vi "Scoring.vi"(4 "Target Up?":bool, 7 "Cluster In":T1, 8 "Hit?":bool, 9 "Falling Edge":bool, 10 "FallingEdge":u32, 11 "RisingEdge":u32) -> (1 "Combo":u32, 2 "Live Score":u32, 3 "Cluster Out":T1)   [LabVIEW 2022 SP3]
uses:
  ShargTypeDef.ctl
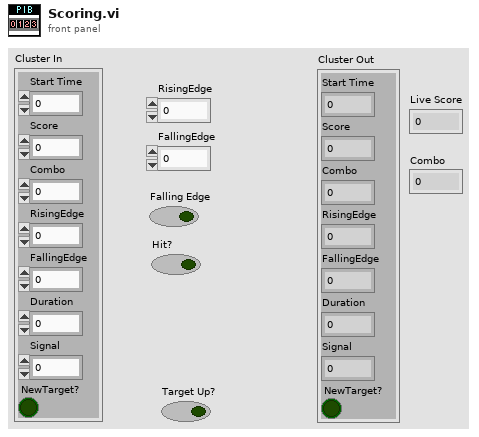
[diagram p1: front panel]
types:
  T1 = typedef "ShargTypeDef.ctl" = cluster{"Start Time":u32, "Score":u32, "Combo":u32, "RisingEdge":u32, "FallingEdge":u32, "Duration":u32, "Signal":i16, "NewTarget?":bool}
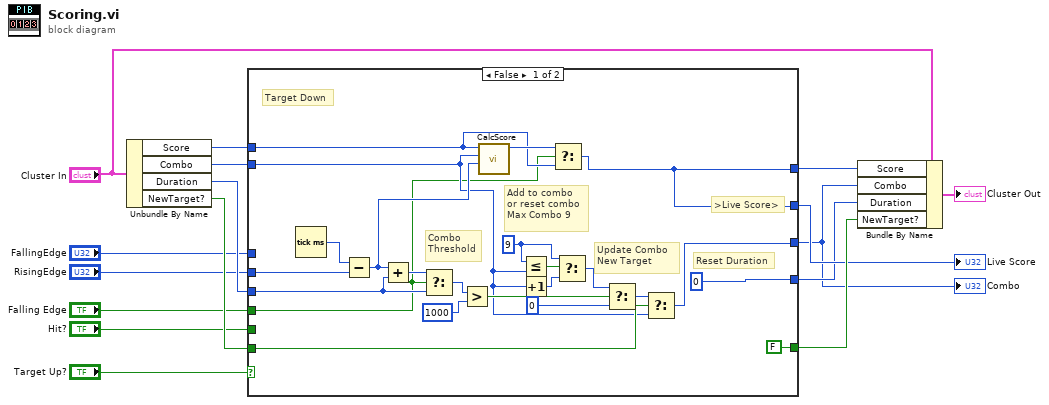
[diagram p0: block diagram]
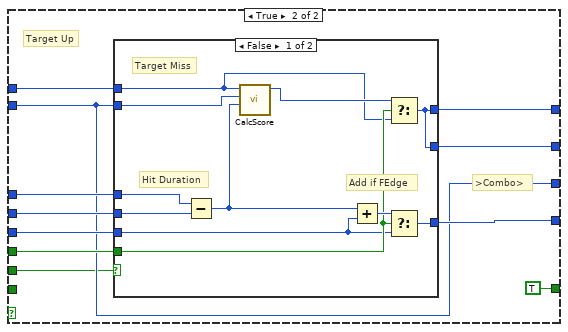
[diagram p2: hidden frame]
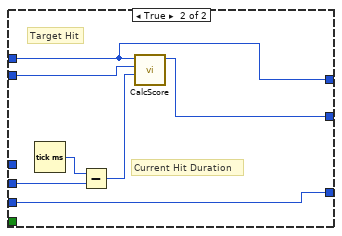
[diagram p3: hidden frame]
diagram:
  n1 = Unbundle By Name("Cluster In") -> ("Score"=w8:u32, "Combo"=w9:u32, "Duration"=w10:u32, "NewTarget?"=w11:bool)
  n2 = case shown="False" "Target Up?" {
    tunnel: "Hit?" -> [_ w40]
    tunnel: "RisingEdge" -> [w31 w45]
    tunnel: "FallingEdge" -> [_ w44]
    tunnel: w10 -> [w18 w43]
    tunnel: [u32 0 ("Duration") w50] -> w14
    tunnel: "Falling Edge" -> [w17 w49]
    tunnel: w9 -> [w25 w42]
    tunnel: [w35 w42] -> w13
    tunnel: [FALSE TRUE] -> w16
    tunnel: w11 -> [w33 _]
    tunnel: w8 -> [w21 w46]
    tunnel: [w23 w47] -> w12
    tunnel: [w23 w41] -> w15
    frame False {
      w24 = u32 9 ("t")
      # ">Live Score>"
      # "Reset Duration"
      # "Update Combo\nNew Target"
      # "Add to combo\nor reset combo\nMax Combo 9"
      # "Combo\nThreshold"
      # "Target Down"
      n3 = Tick Count (ms)() -> (millisecond timer value=w30:u32)
      n4 = Subtract(x=w30, y=w31) -> (x-y=w29:u32)
      n5 = Add(x=w29, y=w18) -> (x+y=w20:u32)
      n6 = Select(t=w20, s=w17, f=w18) -> (s? t:f=w19:u32)
      n7 = Greater?(x=w19, y=u32 1000) -> (0:w37:bool)
      n8 = call "CalcScore.vi"(">HitTime>"=w29, "Combo"=w25, "OldScore"=w21) -> ("NewScore"=w22:u32)  [unwired: 8 in]
      n9 = Less Or Equal?(x=w24, y=w25) -> (x <= y?=w26:bool)
      n10 = Increment(x=w25) -> (x+1=w27:u32)
      n11 = Select(t=w22, s=w17, f=w21) -> (s? t:f=w23:u32)
      n12 = Select(t=w24, s=w26, f=w27) -> (s? t:f=w28:u32)
      n13 = Select(t=w28, s=w37, f=u32 0) -> (s? t:f=w34:u32)
      n14 = Select(t=w34, s=w33, f=w25) -> (s? t:f=w35:u32)
    }
    frame True {
      # ">Combo>"
      # "Target Up"
      n15 = case shown="False" w40 {
        tunnel: w45 -> [w60 w67]
        tunnel: w43 -> [w55 w66]
        tunnel: w44 -> [w61 _]
        tunnel: [w57 w66] -> w50
        tunnel: w49 -> [w56 _]
        tunnel: w46 -> [w51 w62]
        tunnel: w42 -> [w53 w64]
        tunnel: [w58 w62] -> w47
        tunnel: [w58 w63] -> w41
        frame False {
          # "Add if FEdge"
          # "Hit Duration"
          # "Target Miss"
          n16 = Subtract(x=w61, y=w60) -> (x-y=w54:u32)
          n17 = call "CalcScore.vi"(">HitTime>"=w54, "Combo"=w53, "OldScore"=w51) -> ("NewScore"=w52:u32)  [unwired: 8 in]
          n18 = Add(x=w54, y=w55) -> (x+y=w59:u32)
          n19 = Select(t=w52, s=w56, f=w51) -> (s? t:f=w58:u32)
          n20 = Select(t=w59, s=w56, f=w55) -> (s? t:f=w57:u32)
        }
        frame True {
          # "Current Hit Duration"
          # "Target Hit"
          n21 = Tick Count (ms)() -> (millisecond timer value=w68:u32)
          n22 = Subtract(x=w68, y=w67) -> (x-y=w65:u32)
          n23 = call "CalcScore.vi"(">HitTime>"=w65, "Combo"=w64, "OldScore"=w62) -> ("NewScore"=w63:u32)  [unwired: 8 in]
        }
      }
    }
  }
  "Live Score" <- w15
  "Combo" <- w13
  n24 = Bundle By Name(cluster="Cluster In", "Score"=w12, "Combo"=w13, "Duration"=w14, "NewTarget?"=w16) -> (→"Cluster Out":T1)
